vi "Test for reachability.vi"(8 "error in (no error)":errorcluster, 10 "must be directly reachable?":bool, 11 "address":refnum<class "IPv4 Network Address.lvclass">) -> (0 "error out":errorcluster, 2 "found?":bool, 3 "address out":refnum<class "Generic Network Address.lvclass">)   [LabVIEW 2020, in "NI_WFCN.lvlib" / "IPv4 Network Address.lvclass"]
doc: "Determine whether the specified address is reachable."
uses:
  <vilib>/net/WFCN/Addressing/IPv4 Network Address/IPv4 Network Address.lvclass
  e:/builds/penguin/labview/branches/2020/dev/dist/vi.lib/net/WFCN/Addressing/Generic Network Address/Generic Network Address.lvclass
  <vilib>/net/WFCN/Addressing/Generic Network Address/Generic Network Address.lvclass
  <vilib>/net/WFCN/Addressing/IPv4 Network Address/IPv4 Network Address.lvclass/IPv4 Network Address.ctl
  <vilib>/net/WFCN/Addressing/IPv4 Network Address/Create from U32.vi
  <vilib>/net/WFCN/Utility/Subnet Mask to CIDR Prefix.vi
  <vilib>/net/WFCN/Utility/To Native Byte Order U32.vi
  <vilib>/net/WFCN/Addressing/IPv4 Network Address/IPv4LL Numeric Address Constant.vi
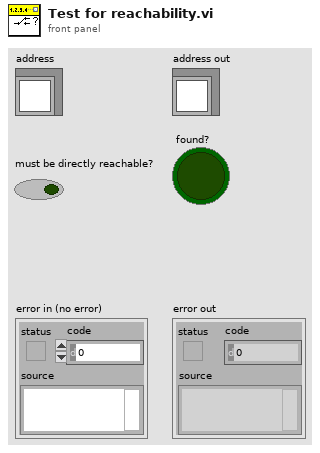
[diagram p1: front panel]
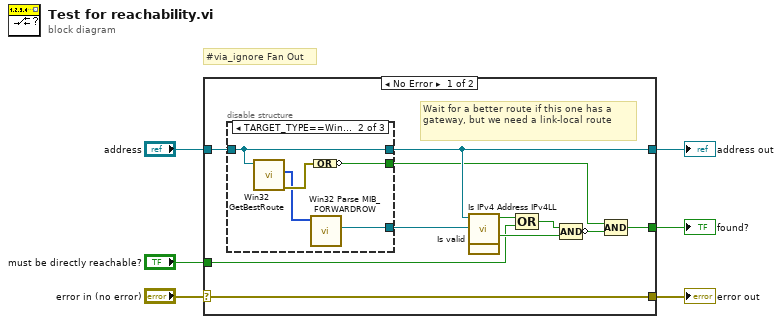
[diagram p0: block diagram]
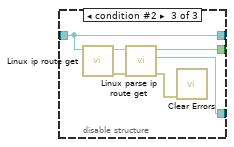
[diagram p3: hidden frame]
diagram:
  # "#via_ignore Fan Out"
  n1 = case shown="No Error" "error in (no error)" {
    selector: "error in (no error)" -> [w7 w30]
    tunnel: [w13 _] -> w6
    tunnel: "address" -> [w17 w31]
    tunnel: [w7 w30] -> w4
    tunnel: [w16 w31] -> w3
    tunnel: "must be directly reachable?" -> [w10 _]
    frame No Error {
      # "Wait for a better route if this one has a gateway, but we need a link-local route"
      n2 = disable-structure shown="TARGET_TYPE==Windows" {
        disable-tunnel: [_ w23 w27] -> w14
        disable-tunnel: w17 -> [w18 w19 w25]
        disable-tunnel: [w18 w19 w25] -> w16
        disable-tunnel: [_ w20 w26] -> w15
        frame condition #0 {
        }
        frame condition #1 (active) {
          n3 = call <vilib>:"Win32 GetBestRoute.vi"("address"=w19) -> ("error out"=w22:errorcluster, "pBestRoute"=w21:u32[])  [unwired: 9 in]
          n4 = call <vilib>:"Win32 Parse MIB_FORWARDROW.vi"("pBestRoute"=w21) -> ("address out"=w20:refnum<class "Generic Network Address.lvclass">)  [unwired: 8 in, 2 out]
          n5 = Compound Arithmetic op=OR(w22) -> (invert w23:bool)
        }
        frame condition #2 {
          n6 = call <vilib>:"Linux ip route get.vi"("address"=w25) -> ("error out"=w29:errorcluster, "ip route get stdout"=w28:string)  [unwired: 8 in, 1 out]
          n7 = call <vilib>:"Linux parse ip route get.vi"("error in (no error)"=w29, "ip route get output"=w28) -> ("error out"=w24:errorcluster, "gw"=w26:refnum<class "Generic Network Address.lvclass">, "route ok?"=w27:bool)  [unwired: 7 in]
          n8 = call <vilib>:"Clear Errors.vi"("error in (no error)"=w24) -> ()  [unwired: 5 in, 2 out]
        }
      }
      n9 = call <vilib>:"Is IPv4 Address IPv4LL.vi"("address"=w16) -> ("IPv4LL?"=w11:bool)  [unwired: 10 in]
      n10 = call-dynamic "Is valid.vi"("address"=w15) -> ("valid?"=w12:bool)  [unwired: 9 in, 1 out]
      n11 = Compound Arithmetic op=OR(w11, w10) -> (w9:bool)
      n12 = Compound Arithmetic op=AND(w9, w12) -> (invert w8:bool)
      n13 = Compound Arithmetic op=AND(w14, w8) -> (w13:bool)
    }
    frame Error {
    }
  }
  "error out" <- w4
  "address out" <- w3
  "found?" <- w6
